vi "Lockin_Vsg_Pubudu.vi"(8 "error in (no error)":errorcluster, 11 "Transport":refnum<class "Transport.lvclass">) -> (0 "error out":errorcluster, 3 "Transport.lvclass":refnum<class "Transport.lvclass">)   [LabVIEW 2019, in "Transport.lvclass"]
uses:
  <userlib>/LevyLab/Transport/Transport/Transport.lvclass
  <userlib>/LevyLab/Transport/Control Experiment/Typedefs/Instruments--cluster.ctl
  <userlib>/LevyLab/Krohn Hite 7008/Instrument.KH7008.lvclass
  <userlib>/LevyLab/Lockin-Multichannel/Instrument.Lockin/Instrument.Lockin.lvclass
  <userlib>/LevyLab/Instrument Framework/Instrument Types/Cryostat/Instrument.Cryostat.lvclass
  <userlib>/LevyLab/Instrument Framework/Instrument Types/CBridge/Instrument.CBridge.lvclass
  <userlib>/LevyLab/Instrument Framework/Instrument Types/Delay Line/Instrument.DelayLine.lvclass
  <userlib>/LevyLab/Instrument Framework/Instrument Types/Strain/Instrument.Strain.lvclass
  <userlib>/LevyLab/Instrument Framework/Instrument Types/VNA/Instrument.VNA.lvclass
  <userlib>/LevyLab/Instrument Framework/Instrument Types/VSource/Instrument.VSource.lvclass
  <userlib>/LevyLab/Transport/Transport/Transport.lvclass/Transport.ctl
  <userlib>/LevyLab/Transport/Control Experiment/Control Experiment.lvclass/Control Experiment.ctl
  <userlib>/LevyLab/Lockin-Multichannel/Instrument.Lockin/Typedefs/Results Type--Enum.ctl
  <userlib>/LevyLab/Lockin-Multichannel/Lockin.DAQ/Typedefs/AO_Channel-Numeric.ctl
  <userlib>/LevyLab/Transport/Control Experiment/Control Experiment.lvclass
  <userlib>/LevyLab/Lockin-Multichannel/Lockin.DAQ/Lockin.DAQ.lvclass
panel:
  in  "Tab Control":enum32{"LockIn Control", "Data", "Other"}(tab)
  out "elapsed time (s)":u32=1660
  in  "Input":i32[](array[numeric])=[21]
  in  "Vmax (end)":dbl=5.0 format="%#_3p"
  in  "Vmin (start)":dbl=-5.0 format="%#_3p"
  in  "dV":dbl=0.025 format="%#_3p"
  in  "Experiment Comments":string="Vbg sweep from  0V to 100V to  -100V to 0V in steps of 0.5V\n\nstripe device:\n\nI+: 11,12,13, current mode, gain: 1000x, shunt resistor : 5kohm \nlead 12: Vac: 125uV, 7Hz, Vdc= 0mV\ndV1: 11-12 voltage mode, gain: 10x, shunt resistor : open \nVbg: 26, 1Gohm resistor\n\nhash device:\n\nI+: 16,17 current mode, gain: 1000x, shunt resistor : 5kohm \nlead 17: Vac:  5mV, 7Hz, Vdc= 0mV\n##lead 20, voltage mode, gain: 10x, shunt resistor : open \ndV1: 16-17 voltage mode, gain: 10x, shunt resistor : open \n##dV1: 16-20 voltage mode, gain: 10x, shunt resistor : open \nVbg: 26, 1Gohm resistor\n\nIn plane gates:\n3,8,15,21: 0V, 100Mohm resistors"
  in  "Experiment Folder":string="14- mega backgate sweep"
  out "T (mK)":dbl=0.001
  in  "wait after setting Vsg (ms)":u32=2000
  in  "Initial wait (ms)":u32=1000
  in  "Sweep":enum16{"Vsg", "Vbg"}(ring)
  in  "cycles (1,2,...)":i32=1 min=1 step=1
  in  "phase":dbl
  out "Field (T)":dbl=-0.0003 format="%#_13g"
  in  "function (ramp)":enum16{"Ramp", "Triangle", "Sine"}(ring)=enum."Triangle"
  in  "set \"Vsg\" to initial value?":bool
  out "time b/w points (ms)":u32=2066
  in  "stop":bool
  out "APD Signal":dbl[](graph)
  out "X Lockins":cluster{dbl[], dbl[]}[](graph)
  out "Y Lockins":cluster{dbl[], dbl[]}[](graph)
  out "G4T":cluster{dbl[], dbl[]}[](graph)
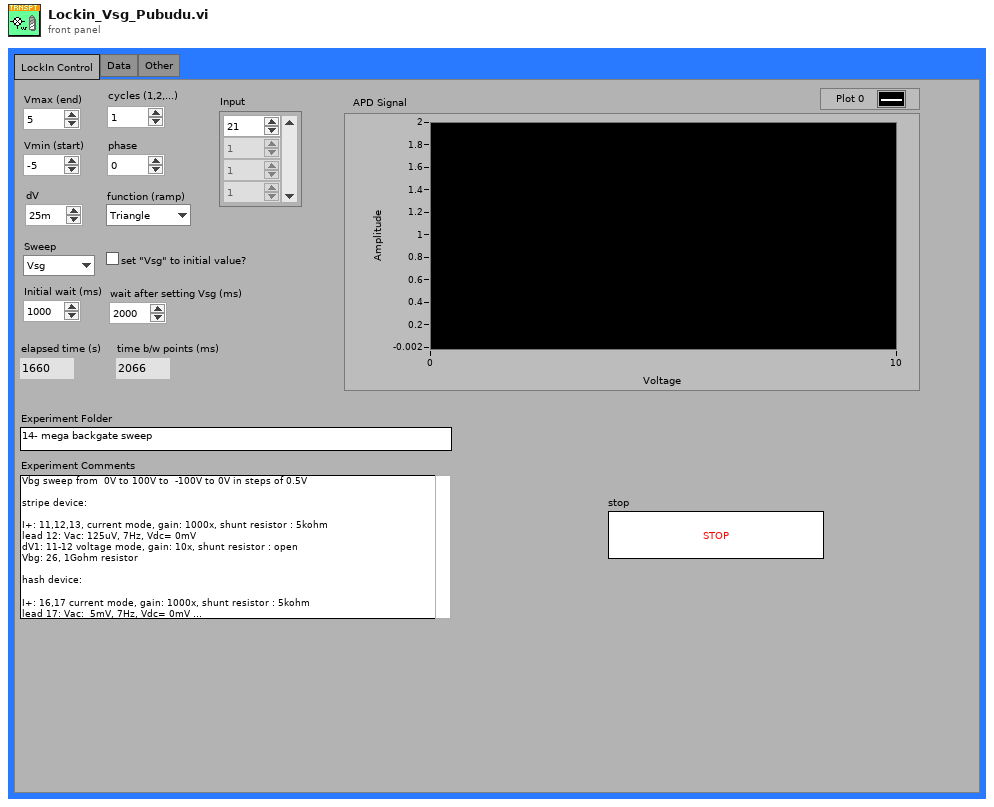
[diagram p1: front panel]
types:
  T1 = enum32{"Invalid", "Standard", "Closed", "Hidden", "Minimized", "Maximized"}
  T2 = enum32{"invalid app kind", "Development System", "Run Time System", "Student Edition", "Embedded LabVIEW", "Evaluation", "Custom"}
  T3 = typedef "Instrument.Lockin.lvclass/Results Type--Enum.ctl" = enum16{"X", "Y", "R", "Theta", "Mean"}
  T4 = typedef "Lockin.DAQ.lvclass/AO_Channel-Numeric.ctl" = i32
  T5 = typedef "Control Experiment.lvclass/Instruments--cluster.ctl" = cluster{"KH7008":refnum<class "Instrument.KH7008.lvclass">[], "Lockin":refnum<class "Instrument.Lockin.lvclass">, "Temperature":refnum<class "Instrument.Cryostat.lvclass">, "Magnet":refnum<class "Instrument.Cryostat.lvclass">, "Rotator":refnum<class "Instrument.Cryostat.lvclass">, "Level":refnum<class "Instrument.Cryostat.lvclass">, "Capacitance Bridge":refnum<class "Instrument.CBridge.lvclass">, "Delay Line":refnum<class "Instrument.DelayLine.lvclass">, "Strain Cell":refnum<class "Instrument.Strain.lvclass">, "VNA":refnum<class "Instrument.VNA.lvclass">, "Voltage Source":refnum<class "Instrument.VSource.lvclass">}
  T6 = cluster{"Core":cluster{"Current VI Reference":refnum<vi>, "Close Panel on Exit?":bool}, "Transport":refnum<class "Transport.lvclass">, "C.E.":refnum<class "Control Experiment.lvclass">, "Instruments":T5, "Sweep Values":dbl[], "Results (Dictionary)":cluster{"key":string, "value":dbl}[], "size":i32, "index":i32, "ms [0]":u32, "ms [i]":u32, "Execution:State":enum32{"Bad", "Idle", "Run top level", "Running"}}
  T7 = enum32{"Bad", "Idle", "Run top level", "Running"}
  T8 = cluster{"Current VI Reference":refnum<vi>, "Close Panel on Exit?":bool}
  T9 = cluster{"I-":i32, "I+":i32, "V1-":i32, "V1+":i32, "I2-":i32, "I2+":i32, "V2-":i32, "V2+":i32}
  T10 = typedef "Lockin.DAQ.lvclass/AO-cluster.ctl" = T11[]
  T11 = typedef "Instrument.Lockin.UI.lvclass/AO Channel--Cluster.ctl" = cluster{"Enable?":bool, "Channel":i32, "Amplitude":dbl, "Offset":dbl, "Frequency":dbl, "Phase":dbl, "Function":T12, "Sweeping?":bool}
  T12 = typedef "Lockin.DAQ.lvclass/Function-enum.ctl" = enum16{"Sine", "Triangle", "Square"}
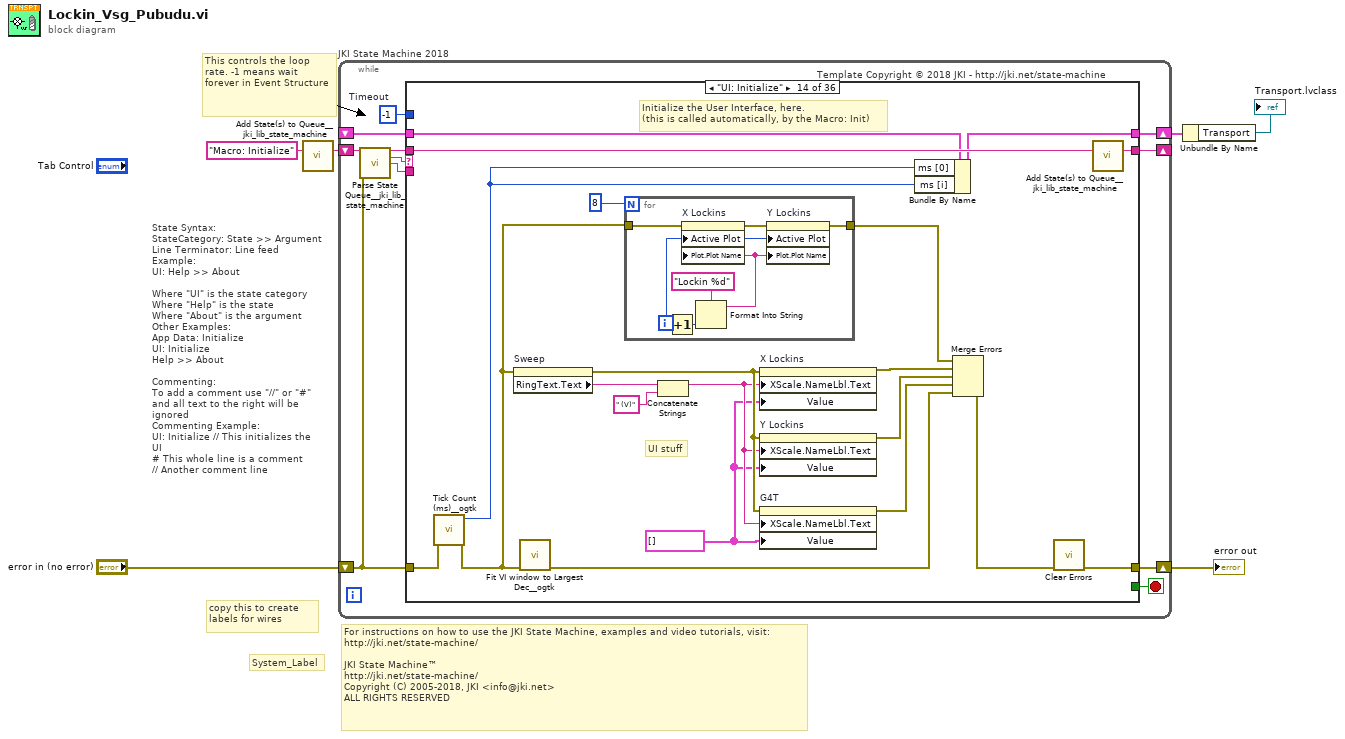
[diagram p0: block diagram]
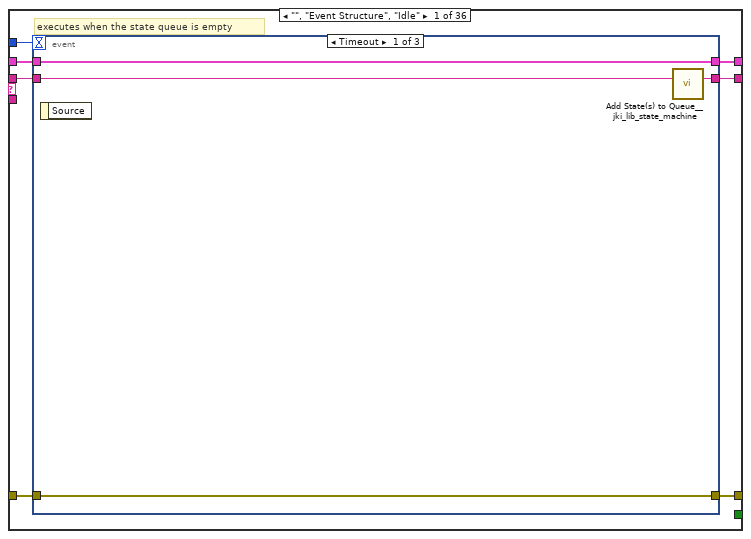
[diagram p2: hidden frame]
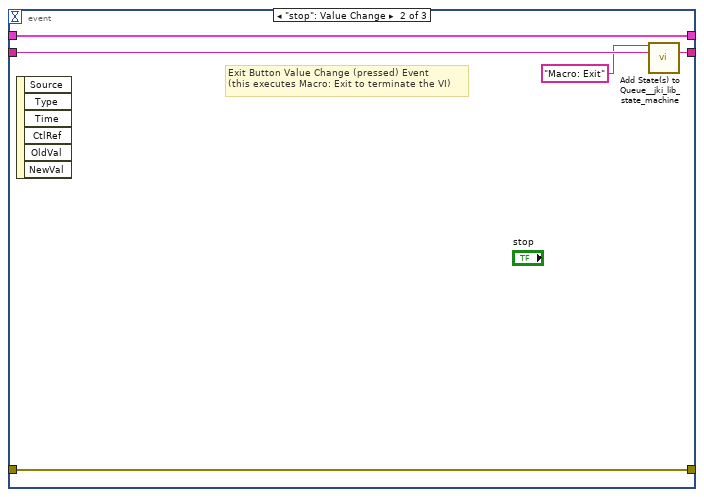
[diagram p3: hidden frame]
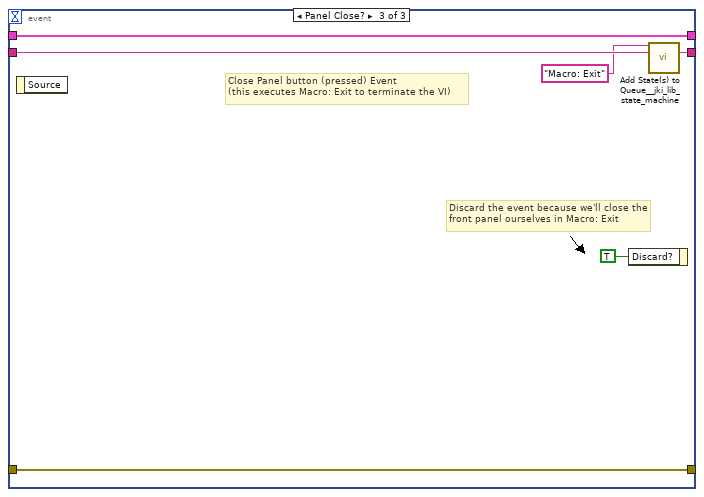
[diagram p4: hidden frame]
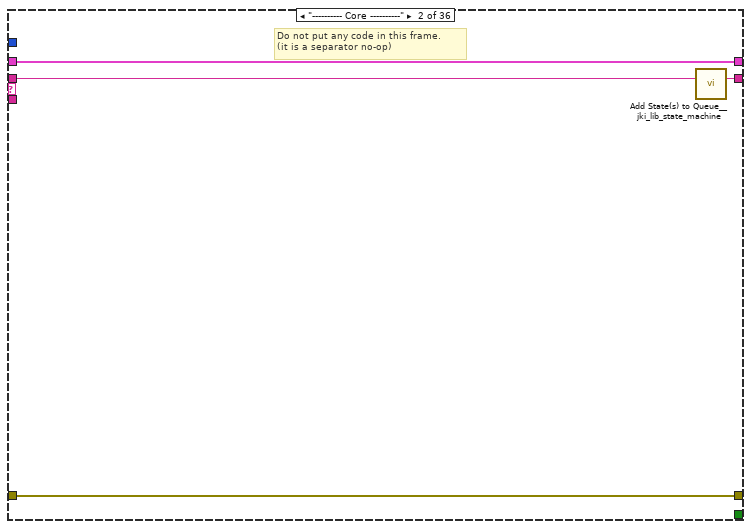
[diagram p5: hidden frame]
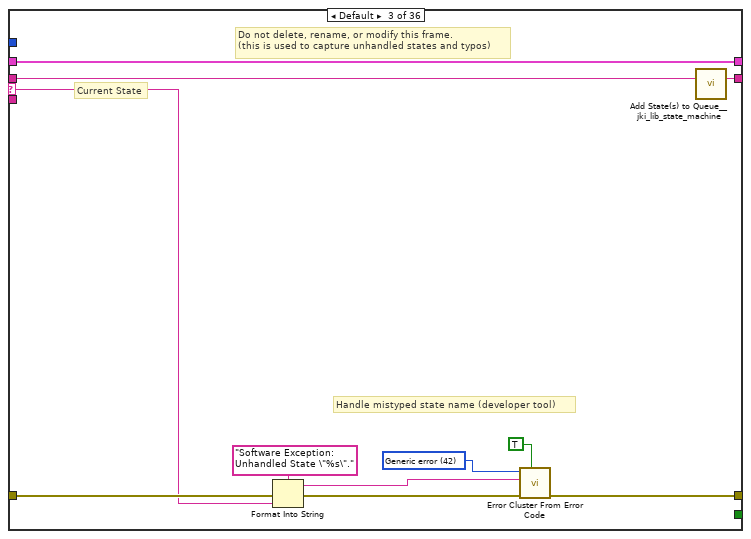
[diagram p6: hidden frame]
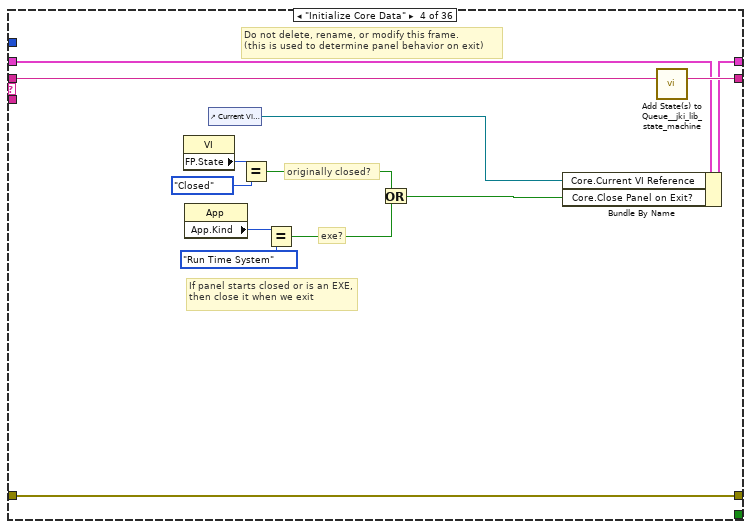
[diagram p7: hidden frame]
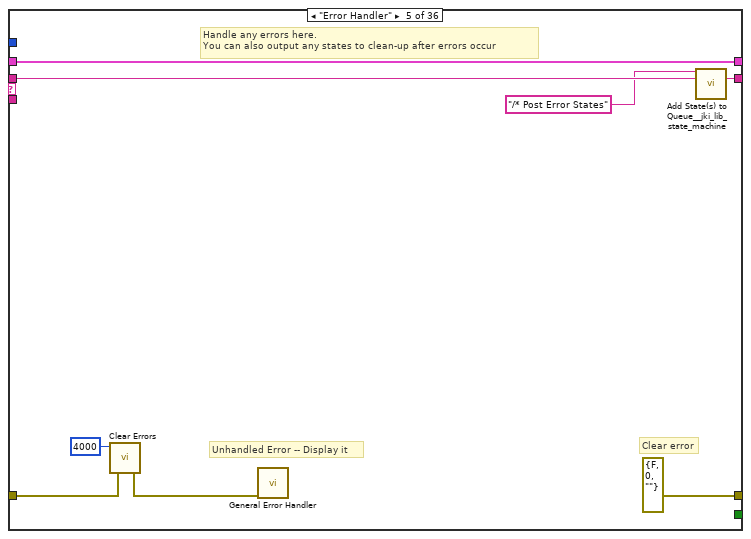
[diagram p8: hidden frame]
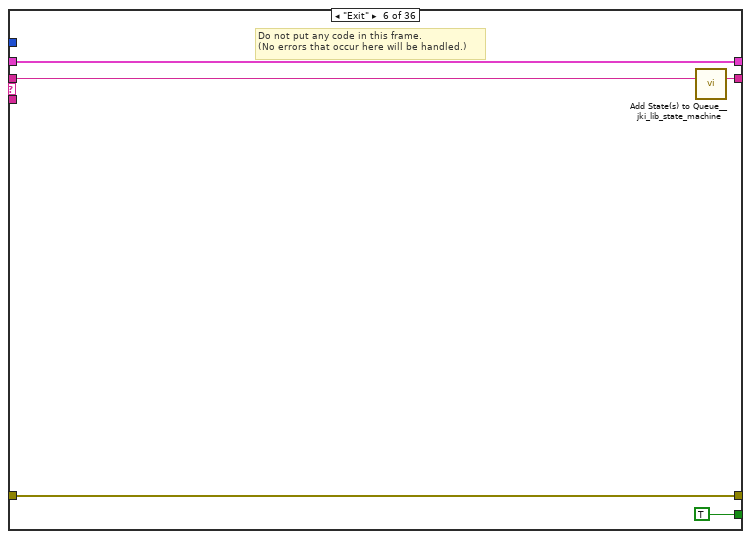
[diagram p9: hidden frame]
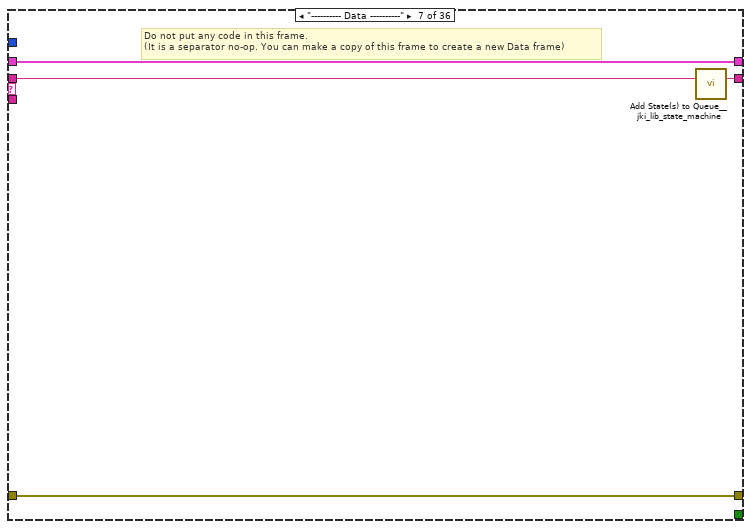
[diagram p10: hidden frame]
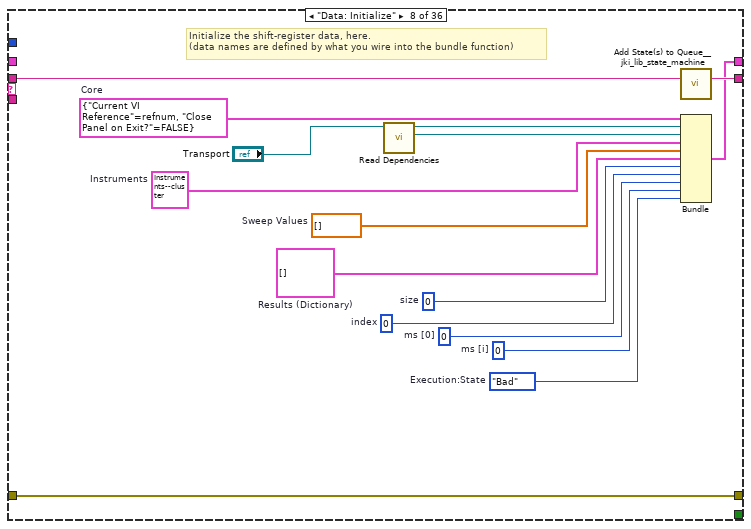
[diagram p11: hidden frame]
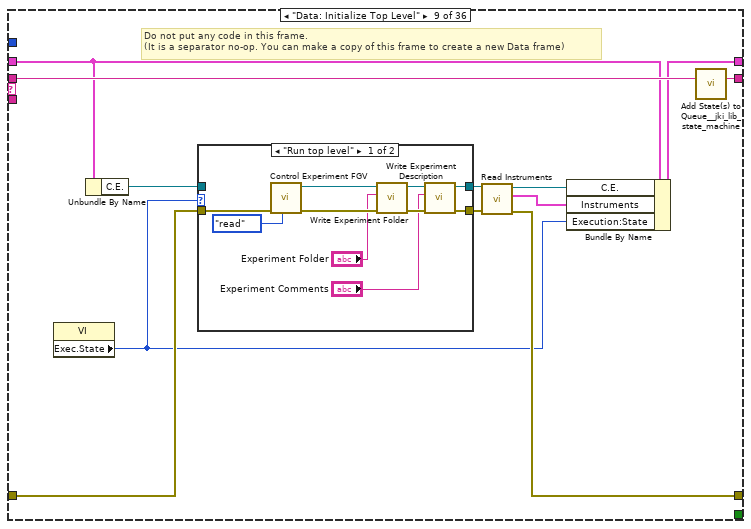
[diagram p12: hidden frame]
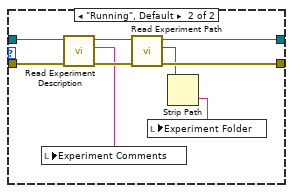
[diagram p13: hidden frame]
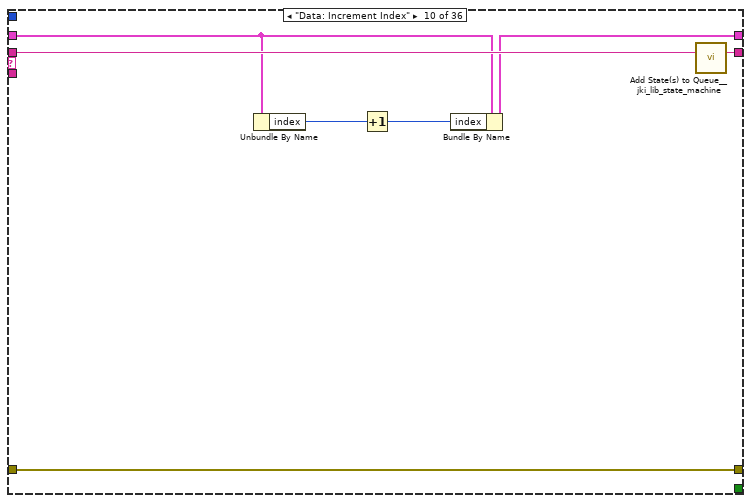
[diagram p14: hidden frame]
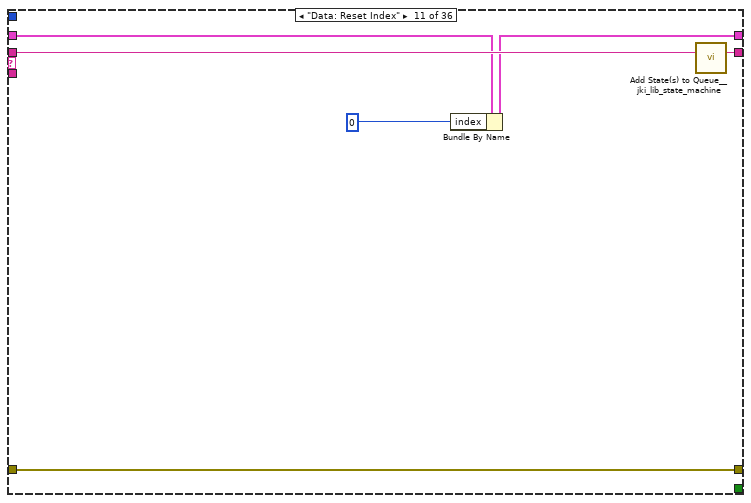
[diagram p15: hidden frame]
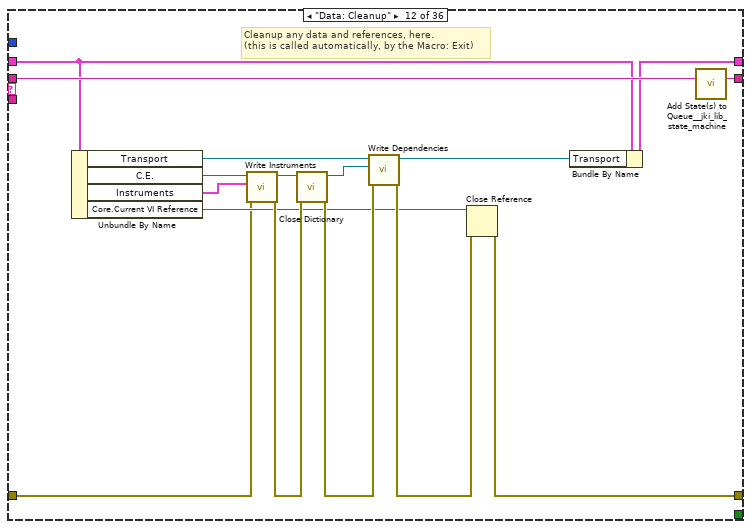
[diagram p16: hidden frame]
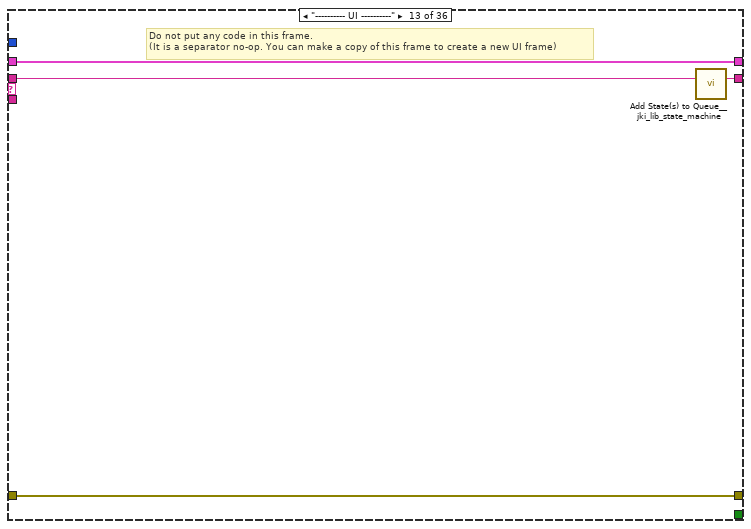
[diagram p17: hidden frame]
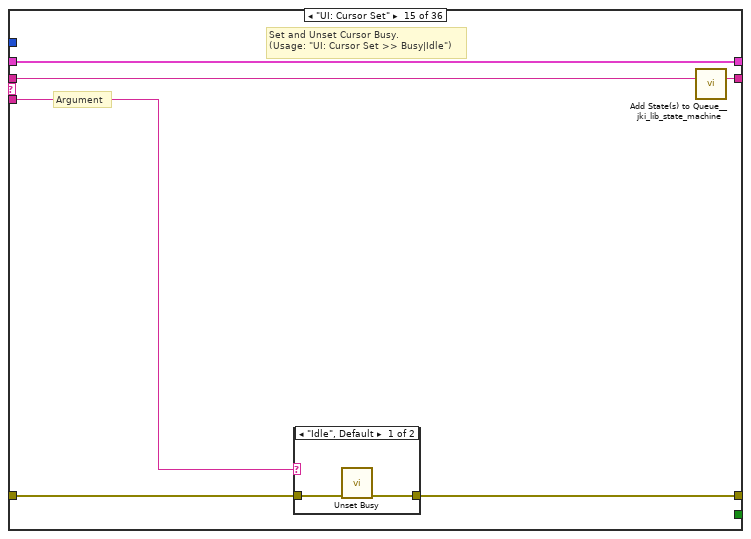
[diagram p18: hidden frame]
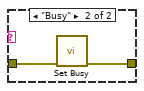
[diagram p19: hidden frame]
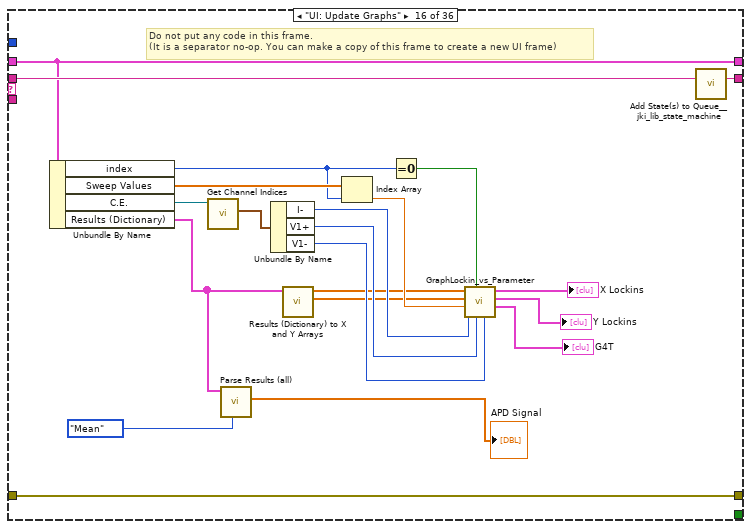
[diagram p20: hidden frame]
diagram:
  # "For instructions on how to use the JKI State Machine, examples and video tutorials, visit:\nhttp://jki.net/state-machine/\n\nJKI State Machine™\nhttp://jki.net/state-machine/\nCopyright (C) 2005-2018, JKI <info@jki.net>\nALL RIGHTS RESERVED"
  # "State Syntax:\nStateCategory: State >> Argument\nLine Terminator: Line feed\nExample:\nUI: Help >> About\n\nWhere \"UI\" is the state category\nWhere \"Help\" is the state\nWhere \"About\" is the argument\nOther Examples:\nApp Data: Initialize\nUI: Initialize\nHelp >> About\n\nCommenting:\nTo add a comment use \"//\" or \"#\" and all text to the right will be ignored\nCommenting Example:\nUI: Initialize // This initializes the UI\n# This whole line is a comment\n// Another comment line"
  # "copy this to create labels for wires"
  # "This controls the loop rate. -1 means wait forever in Event Structure"
  # "System_Label"
  n1 = call <vilib>:"Add State(s) to Queue__jki_lib_state_machine.vi"("State(s) in (\"\")"="Macro: Initialize") -> ("States Out"=w6:string)  [unwired: 14 in]
  n2 = while "JKI State Machine 2018" {
    shift-right: [w10] -> w4
    shift-left: _ -> [w9]
    shift-right: [w13] -> w2
    shift-left: "error in (no error)" -> [w7]
    shift-right: [w12] -> _
    shift-left: w6 -> [w14]
    stop <- w11 stop-if-true
    w8 = -1  # Timeout
    # "Template Copyright © 2018 JKI - http://jki.net/state-machine"
    n3 = call <vilib>:"Parse State Queue__jki_lib_state_machine.vi"("State Queue"=w14, "Error In (no error)"=w7) -> ("Remaining States"=w16:string, "Current State"=w17:string, "Arguments"=w15:string)  [unwired: 11 in]
    n4 = case shown="\"UI: Initialize\"" w17 {
      selector: w17 -> [_ _ w44 _ _ _ _ _ _ _ _ _ _ _ _ _ _ _ _ _ _ _ _ _ _ _ _ _ _ _ _ _ _ _ _ _]
      tunnel: w16 -> [w24 w43 w48 w67 w75 w80 w84 w100 w112 w138 w144 w160 w164 w184 w197 w222 w235 w242 w311 w316 w338 w348 w352 w376 w388 w395 w409 w451 w464 w477 w490 w508 w541 w545 w549 w559]
      tunnel: w15 -> [_ _ _ _ _ _ _ _ _ _ _ _ _ _ w192 _ _ w236 _ _ _ _ _ _ _ _ _ _ _ _ _ _ _ _ _ _]
      tunnel: w9 -> [w22 w40 w46 w60 w72 w78 w81 _ w103 w132 w141 w148 w161 w168 w195 w205 w230 w238 w308 w314 w331 w345 w349 w364 w385 w391 w399 w448 w460 w474 w485 w503 w537 w542 w546 w552]
      tunnel: [w21 w41 w50 w64 errorcluster {"status"=FALSE, "code"=0, "source"=""} ("error out") w77 w82 w97 w104 w136 w142 w145 w162 w173 w193 w220 w224 w239 w309 w312 w336 w346 w350 w354 w386 w392 w403 w449 w456 w468 w481 w499 w532 w543 w547 w556] -> w13
      tunnel: w7 -> [w20 w41 w49 w64 w69 w77 w82 w97 w105 w136 w142 w146 w162 w170 w194 w220 w232 w240 w309 w312 w336 w346 w350 w361 w386 w393 w402 w449 w461 w472 w482 w506 w533 w543 w547 w555]
      tunnel: [w23 w42 w47 w66 w74 w79 w83 w99 w111 w137 w143 w159 w163 w183 w196 w221 w234 w241 w310 w315 w337 w347 w351 w375 w387 w394 w408 w450 w463 w476 w489 w507 w540 w544 w548 w558] -> w12
      tunnel: [_ _ _ _ _ TRUE _ _ _ _ _ _ _ _ _ _ _ _ _ _ _ _ _ _ _ _ _ _ _ _ _ _ _ _ _ _] -> w11
      tunnel: [w19 w40 w46 w65 w72 w78 w81 w98 w102 w135 w140 w147 w161 w167 w195 w205 w229 w238 w308 w314 w331 w345 w349 w367 w385 w391 w400 w448 w459 w473 w484 w504 w538 w542 w546 w551] -> w10
      tunnel: w8 -> [w18 _ _ _ _ _ _ _ _ _ _ _ _ _ _ _ _ _ _ _ _ _ _ _ _ _ _ _ _ _ _ _ _ _ _ _]
      frame "", "Event Structure", "Idle" {
        # "executes when the state queue is empty"
        n5 = event shown="[0] Timeout" {
          selector: _ -> [_ _ _]
          dyn-events: _ -> [_ _ _]
          timeout: w18 -> [_ _ _]
          tunnel: w24 -> [w28 w33 w39]
          tunnel: [w27 w32 w38] -> w23
          tunnel: w22 -> [w25 w30 w36]
          tunnel: [w26 w31 w37] -> w21
          tunnel: w20 -> [w26 w31 w37]
          tunnel: [w25 w30 w36] -> w19
          event Timeout {
            n6 = event-data() -> ()  [unwired: 1 in, 1 out]
            n7 = call <vilib>:"Add State(s) to Queue__jki_lib_state_machine.vi"("State(s) in (\"\")"=w28) -> ("States Out"=w27:string)  [unwired: 14 in]
          }
          event "stop": Value Change {
            # "Exit Button Value Change (pressed) Event\n(this executes Macro: Exit to terminate the VI)"
            n8 = event-data() -> ()  [unwired: 1 in, 6 out]
            n9 = call <vilib>:"Add State(s) to Queue__jki_lib_state_machine.vi"("State(s) in Front (\"\")"="Macro: Exit", "State(s) in (\"\")"=w33) -> ("States Out"=w32:string)  [unwired: 13 in]
          }
          event Panel Close? {
            # "Discard the event because we'll close the front panel ourselves in Macro: Exit"
            # "Close Panel button (pressed) Event\n(this executes Macro: Exit to terminate the VI)"
            n10 = event-data() -> ()  [unwired: 1 in, 1 out]
            n11 = event-data("Discard?"=TRUE) -> ()  [unwired: 1 in, 1 out]
            n12 = call <vilib>:"Add State(s) to Queue__jki_lib_state_machine.vi"("State(s) in Front (\"\")"="Macro: Exit", "State(s) in (\"\")"=w39) -> ("States Out"=w38:string)  [unwired: 13 in]
          }
        }
      }
      frame "---------- Core ----------" {
        # "Do not put any code in this frame.\n(it is a separator no-op)"
        n13 = call <vilib>:"Add State(s) to Queue__jki_lib_state_machine.vi"("State(s) in (\"\")"=w43) -> ("States Out"=w42:string)  [unwired: 14 in]
      }
      frame Default {
        w53 = 42 items=["No error", "Argument error", "Memory is full", "Out of zone", "End of file", "File already open", "Generic file I/O error", "File not found", "File permission error", "Disk is full", "Duplicate path", "Too many files open", "System feature not enabled", "Resource file not found", "Cannot add resource", "Resource not found", "Image not found", "Image memory error", "Pen does not exist", "Config type invalid", "Config token not found", "Config parse error", "Config memory error", "Bad external code format", "Bad external code offset", "External code not present", "Null window", "Destroy window error", "Null menu", "Print aborted", "Bad print record", "Print driver error", "Windows error during printing", "Memory error during printing", "Print dialog error", "Generic print error", "Invalid device refnum", "Device not found", "Device parameter error", "Device unit error", "Cannot open device", "Device call aborted", "Generic error", "Cancelled by user", "Object ID too low", "Object ID too high", "Object not in heap", "Unknown heap", "Unknown object (invalid DefProc)", "Unknown object (DefProc not in table)", "Message out of range", "Invalid (null) method", "Unknown message", "Manager call not supported", "Bad address", "Network operation in progress", "Network operation timed out", "Connection is busy", "Network attribute not supported", "Network error", "Address in use", "System out of memory", "Connection aborted", "Connection refused", "Not connected", "Already connected", "Connection closed", "Initialization error (interapplication manager)", "Bad occurrence", "Wait on unbound occurrence handler", "Occurrence queue overflow", "Datalog type conflict", "Unused", "Unrecognized type (interapplication manager)", "Memory corrupt", "Failed to make temporary DLL", "Old CIN version", "Drag socket not found", "Failed to load drop-object", "Failed to register OLE object", "Failed to release OLE object", "Format specifier type mismatch", "Unknown format specifier", "Too few format specifiers", "Too many format specifiers", "Scan failed", "Newer CIN version", "Error converting to variant", "Runtime menu error", "Password tampered", "Variant attribute not found", "Incompatible variant data type", "Event data is not available", "Event Store is not present", "Occurrence is not found", "Event Queue is not created", "Event info is not available", "Refnum passed is NULL", "Error retrieving Class GUID", "Error retrieving CoClass GUID", "Error retrieving TypeLib GUID.", "Bad built application magic bytes.", "Specific driver is different from the specific driver associated with the Logical Name.", "There is no session opened to the class driver.", "Max Error", "MAX - Error with config objects", "MAX - Error loading configuration", "MAX - Group not supported"]
        # "Current State"
        # "Do not delete, rename, or modify this frame.\n(this is used to capture unhandled states and typos)"
        # "Handle mistyped state name (developer tool)"
        n14 = Format Into String(format string="Software Exception: Unhandled State \"%s\"." ("message"), error in=w49, w44) -> (resulting string=w52:string, error out=w51:errorcluster)  [unwired: 1 in]
        n15 = call <vilib>:"Error Cluster From Error Code.vi"("show call chain? (False)"=TRUE, "error in (no error)"=w51, "error message (\"\")"=w52, "error code (0)"=w53) -> ("error out"=w50:errorcluster)  [unwired: 5 in]
        n16 = call <vilib>:"Add State(s) to Queue__jki_lib_state_machine.vi"("State(s) in (\"\")"=w48) -> ("States Out"=w47:string)  [unwired: 14 in]
      }
      frame "Initialize Core Data" {
        # "Do not delete, rename, or modify this frame.\n(this is used to determine panel behavior on exit)"
        # "originally closed?"
        # "exe?"
        # "If panel starts closed or is an EXE, then close it when we exit"
        n17 = property class="VI"() -> ("FP.State"=w57:T1)  [unwired: 2 in, 2 out]
        n18 = property class="App"() -> ("App.Kind"=w63:T2)  [unwired: 2 in, 2 out]
        n19 = control-ref of="Current VI Reference"() -> (w58:refnum<vi>)
        n20 = Equal?(x=w57, y=T1."Closed" ("Front Panel Window:State")) -> (x = y?=w55:bool)
        n21 = Equal?(x=w63, y=T2."Run Time System" ("Application:Kind")) -> (x = y?=w61:bool)
        n22 = Or(x=w55, y=w61) -> (x .or. y?=w59:bool)
        n23 = Bundle By Name(cluster=w60, "Core.Current VI Reference"=w58, "Core.Close Panel on Exit?"=w59) -> (w65:T6)
        n24 = call <vilib>:"Add State(s) to Queue__jki_lib_state_machine.vi"("State(s) in (\"\")"=w67) -> ("States Out"=w66:string)  [unwired: 14 in]
      }
      frame "Error Handler" {
        # "Unhandled Error -- Display it"
        # "Handle any errors here.\nYou can also output any states to clean-up after errors occur"
        # "Clear error"
        n25 = call <vilib>:"Clear Errors.vi"("error in (no error)"=w69, "specific error code to clear (0: all)"=4000) -> ("error out"=w68:errorcluster)  [unwired: 4 in, 1 out]
        n26 = call <vilib>:"General Error Handler.vi"("error in (no error)"=w68) -> ()  [unwired: 10 in, 5 out]
        n27 = call <vilib>:"Add State(s) to Queue__jki_lib_state_machine.vi"("State(s) in Front (\"\")"="/* Post Error States", "State(s) in (\"\")"=w75) -> ("States Out"=w74:string)  [unwired: 13 in]
      }
      frame "Exit" {
        # "Do not put any code in this frame.\n(No errors that occur here will be handled.)"
        n28 = call <vilib>:"Add State(s) to Queue__jki_lib_state_machine.vi"("State(s) in (\"\")"=w80) -> ("States Out"=w79:string)  [unwired: 14 in]
      }
      frame "---------- Data ----------" {
        # "Do not put any code in this frame.\n(It is a separator no-op. You can make a copy of this frame to create a new Data frame)"
        n29 = call <vilib>:"Add State(s) to Queue__jki_lib_state_machine.vi"("State(s) in (\"\")"=w84) -> ("States Out"=w83:string)  [unwired: 14 in]
      }
      frame "Data: Initialize" {
        w85 = cluster{"key":string, "value":dbl}[] []  # Results (Dictionary)
        w89 = T7."Bad"  # Execution:State
        w90 = 0  # size
        w91 = u32 0  # ms [i]
        w92 = u32 0  # ms [0]
        w93 = 0  # index
        w94 = dbl[] []  # Sweep Values
        w95 = T5 {"KH7008"=[], "Lockin"=refnum, "Temperature"=refnum, "Magnet"=refnum, "Rotator"=refnum, "Level"=refnum, "Capacitance Bridge"=refnum, "Delay Line"=refnum, "Strain Cell"=refnum, "VNA"=refnum, "Voltage Source"=refnum}  # Instruments
        w96 = T8 {"Current VI Reference"=refnum, "Close Panel on Exit?"=FALSE}  # Core
        # "Initialize the shift-register data, here.\n(data names are defined by what you wire into the bundle function)"
        n30 = call <userlib>:"Read Dependencies.vi"("Transport"="Transport") -> ("C.E."=w87:refnum<class "Control Experiment.lvclass">, "Transport"=w86:refnum<class "Transport.lvclass">)  [unwired: 8 in, 1 out]
        n31 = call <vilib>:"Add State(s) to Queue__jki_lib_state_machine.vi"("State(s) in (\"\")"=w100) -> ("States Out"=w99:string)  [unwired: 14 in]
        n32 = Bundle("Core"=w96, "Transport"=w86, "C.E."=w87, "Instruments"=w95, "Sweep Values"=w94, "Results (Dictionary)"=w85, "size"=w90, "index"=w93, "ms [0]"=w92, "ms [i]"=w91, "Execution:State"=w89) -> (w98:T6)  [unwired: 1 in]
      }
      frame "Data: Initialize Top Level" {
        # "Do not put any code in this frame.\n(It is a separator no-op. You can make a copy of this frame to create a new Data frame)"
        n33 = property class="VI"() -> ("Exec.State"=w101:T7)  [unwired: 2 in, 2 out]
        n34 = Unbundle By Name(w103) -> ("C.E."=w106:refnum<class "Control Experiment.lvclass">)
        n35 = case shown="\"Run top level\"" w101 {
          tunnel: w105 -> [w122 w130]
          tunnel: [w117 w126] -> w107
          tunnel: [w116 w127] -> w108
          tunnel: w106 -> [_ w131]
          frame "Run top level" {
            n36 = call <userlib>:"Control Experiment FGV.vi"("Function"=enum16{"read", "write"}."read", "error in (no error)"=w122) -> ("error out"=w120:errorcluster, "Control Experiment.lvclass out"=w121:refnum<class "Control Experiment.lvclass">)  [unwired: 8 in]
            n37 = call <userlib>:"Write Experiment Folder.vi"("error in (no error)"=w120, "Experiment Folder"="Experiment Folder", "Control Experiment in"=w121) -> ("error out"=w118:errorcluster, "Control Experiment out"=w119:refnum<class "Control Experiment.lvclass">)  [unwired: 7 in]
            n38 = call <userlib>:"Write Experiment Description.vi"("error in (no error)"=w118, "Experiment Description"="Experiment Comments", "Control Experiment in"=w119) -> ("error out"=w117:errorcluster, "Control Experiment out"=w116:refnum<class "Control Experiment.lvclass">)  [unwired: 7 in]
          }
          frame "Running", Default {
            n39 = call <userlib>:"Read Experiment Description.vi"("error in (no error)"=w130, "Control Experiment in"=w131) -> ("error out"=w129:errorcluster, "Experiment Description"=w124:string, "Control Experiment out"=w128:refnum<class "Control Experiment.lvclass">)  [unwired: 7 in]
            n40 = local write "Experiment Comments"(w124) -> ()
            n41 = call <userlib>:"Read Experiment Path.vi"("error in (no error)"=w129, "Control Experiment in"=w128) -> ("error out"=w126:errorcluster, "Experiment Path"=w125:path, "Control Experiment out"=w127:refnum<class "Control Experiment.lvclass">)  [unwired: 7 in]
            n42 = Strip Path(path=w125) -> (name=w123:string)  [unwired: 1 out]
            n43 = local write "Experiment Folder"(w123) -> ()
          }
        }
        n44 = call <userlib>:"Read Instruments.vi"("error in (no error)"=w107, "Control Experiment in"=w108) -> ("error out"=w104:errorcluster, "Instruments"=w110:T5, "Control Experiment out"=w109:refnum<class "Control Experiment.lvclass">)  [unwired: 7 in]
        n45 = Bundle By Name(cluster=w103, "C.E."=w109, "Instruments"=w110, "Execution:State"=w101) -> (w102:T6)
        n46 = call <vilib>:"Add State(s) to Queue__jki_lib_state_machine.vi"("State(s) in (\"\")"=w112) -> ("States Out"=w111:string)  [unwired: 14 in]
      }
      frame "Data: Increment Index" {
        n47 = Unbundle By Name(w132) -> ("index"=w134:i32)
        n48 = Increment(x=w134) -> (x+1=w133:i32)
        n49 = Bundle By Name(cluster=w132, "index"=w133) -> (w135:T6)
        n50 = call <vilib>:"Add State(s) to Queue__jki_lib_state_machine.vi"("State(s) in (\"\")"=w138) -> ("States Out"=w137:string)  [unwired: 14 in]
      }
      frame "Data: Reset Index" {
        n51 = Bundle By Name(cluster=w141, "index"=0) -> (w140:T6)
        n52 = call <vilib>:"Add State(s) to Queue__jki_lib_state_machine.vi"("State(s) in (\"\")"=w144) -> ("States Out"=w143:string)  [unwired: 14 in]
      }
      frame "Data: Cleanup" {
        # "Cleanup any data and references, here.\n(this is called automatically, by the Macro: Exit)"
        n53 = Unbundle By Name(w148) -> ("Transport"=w157:refnum<class "Transport.lvclass">, "C.E."=w155:refnum<class "Control Experiment.lvclass">, "Instruments"=w153:T5, "Core.Current VI Reference"=w149:refnum<vi>)
        n54 = call <userlib>:"Write Instruments.vi"("error in (no error)"=w146, "Instruments"=w153, "Control Experiment in"=w155) -> ("error out"=w152:errorcluster, "Control Experiment out"=w154:refnum<class "Control Experiment.lvclass">)  [unwired: 7 in]
        n55 = call <userlib>:"Close Dictionary.vi"("error in (no error)"=w152, "Control Experiment in"=w154) -> ("error out"=w151:errorcluster, "Control Experiment out"=w156:refnum<class "Control Experiment.lvclass">)  [unwired: 8 in]
        n56 = call <userlib>:"Write Dependencies.vi"("error in (no error)"=w151, "Control Experiment"=w156, "Transport in"=w157) -> ("error out"=w150:errorcluster, "Transport out"=w158:refnum<class "Transport.lvclass">)  [unwired: 7 in]
        n57 = Close Reference(reference=w149, error in (no error)=w150) -> (error out=w145:errorcluster)
        n58 = Bundle By Name(cluster=w148, "Transport"=w158) -> (w147:T6)
        n59 = call <vilib>:"Add State(s) to Queue__jki_lib_state_machine.vi"("State(s) in (\"\")"=w160) -> ("States Out"=w159:string)  [unwired: 14 in]
      }
      frame "---------- UI ----------" {
        # "Do not put any code in this frame.\n(It is a separator no-op. You can make a copy of this frame to create a new UI frame)"
        n60 = call <vilib>:"Add State(s) to Queue__jki_lib_state_machine.vi"("State(s) in (\"\")"=w164) -> ("States Out"=w163:string)  [unwired: 14 in]
      }
      frame "UI: Initialize" {
        w165 = cluster{dbl[], dbl[]}[] [] ("G4T")
        # "UI stuff"
        # "Initialize the User Interface, here.\n(this is called automatically, by the Macro: Init)"
        n61 = call <userlib>:"Tick Count (ms)__ogtk.vi"("error in (no error)"=w170) -> ("error out"=w169:errorcluster, "millisecond timer value"=w166:u32)  [unwired: 9 in]
        n62 = property on="Sweep" class="Enum (strict)"(error in=w169) -> (error out=w178:errorcluster, "RingText.Text"=w176:string)  [unwired: 1 in, 1 out]
        n63 = call <userlib>:"Fit VI window to Largest Dec__ogtk.vi"("error in (no error)"=w169) -> ("error out"=w172:errorcluster)  [unwired: 5 in, 1 out]
        n64 = for {
          N: 8 -> [_]
          tunnel: [w185] -> w179
          tunnel: w169 -> [w190]
          i -> [w188]
          n65 = Increment(x=w188) -> (x+1=w186:i32)
          n66 = Format Into String(format string="Lockin %d", w186) -> (resulting string=w189:string)  [unwired: 2 in, 1 out]
          n67 = property on="X Lockins" class="XYGraph (strict)"(error in=w190, "Active Plot"=w188, "Plot.Plot Name"=w189) -> (error out=w187:errorcluster)  [unwired: 1 in, 1 out]
          n68 = property on="Y Lockins" class="XYGraph (strict)"(error in=w187, "Active Plot"=w188, "Plot.Plot Name"=w189) -> (error out=w185:errorcluster)  [unwired: 1 in, 1 out]
        }
        n69 = Concatenate Strings(w176, " (V)" ("string")) -> (w177:string)
        n70 = property on="X Lockins" class="XYGraph (strict)"(error in=w178, "XScale.NameLbl.Text"=w177, "Value"=w165) -> (error out=w180:errorcluster)  [unwired: 1 in, 1 out]
        n71 = property on="Y Lockins" class="XYGraph (strict)"(error in=w178, "XScale.NameLbl.Text"=w177, "Value"=w165) -> (error out=w181:errorcluster)  [unwired: 1 in, 1 out]
        n72 = property on="G4T" class="XYGraph (strict)"(error in=w178, "XScale.NameLbl.Text"=w177, "Value"=w165) -> (error out=w182:errorcluster)  [unwired: 1 in, 1 out]
        n73 = Bundle By Name(cluster=w168, "ms [0]"=w166, "ms [i]"=w166) -> (w167:T6)
        n74 = Merge Errors(w179, w180, w181, w182, w172) -> (w171:errorcluster)
        n75 = call <vilib>:"Clear Errors.vi"("error in (no error)"=w171) -> ("error out"=w173:errorcluster)  [unwired: 5 in, 1 out]
        n76 = call <vilib>:"Add State(s) to Queue__jki_lib_state_machine.vi"("State(s) in (\"\")"=w184) -> ("States Out"=w183:string)  [unwired: 14 in]
      }
      frame "UI: Cursor Set" {
        # "Argument"
        # "Set and Unset Cursor Busy.\n(Usage: \"UI: Cursor Set >> Busy|Idle\")"
        n77 = case shown="\"Idle\", Default" w192 {
          tunnel: w194 -> [w199 w201]
          tunnel: [w198 w200] -> w193
          frame "Idle", Default {
            n78 = call <vilib>:"Unset Busy.vi"("error in (no error)"=w199) -> ("error out"=w198:errorcluster)  [unwired: 10 in]
          }
          frame "Busy" {
            n79 = call <vilib>:"Set Busy.vi"("error in (no error)"=w201) -> ("error out"=w200:errorcluster)  [unwired: 9 in, 1 out]
          }
        }
        n80 = call <vilib>:"Add State(s) to Queue__jki_lib_state_machine.vi"("State(s) in (\"\")"=w197) -> ("States Out"=w196:string)  [unwired: 14 in]
      }
      frame "UI: Update Graphs" {
        # "Do not put any code in this frame.\n(It is a separator no-op. You can make a copy of this frame to create a new UI frame)"
        n81 = Unbundle By Name(w205) -> ("index"=w208:i32, "Sweep Values"=w211:dbl[], "C.E."=w218:refnum<class "Control Experiment.lvclass">, "Results (Dictionary)"=w204:cluster{"key":string, "value":dbl}[])
        n82 = call <userlib>:"Get Channel Indices.vi"("Control Experiment in"=w218) -> ("Indices"=w217:T9)  [unwired: 8 in, 2 out]
        n83 = call <userlib>:"Parse Results (all).vi"("Type"=Results_Type--Enum."Mean", "Results (Dictionary)"=w204) -> ("Data"=→"APD Signal":dbl[])  [unwired: 6 in, 3 out]
        n84 = Unbundle By Name(w217) -> ("I-"=w214:i32, "V1+"=w216:i32, "V1-"=w215:i32)
        n85 = call <userlib>:"Results (Dictionary) to X and Y Arrays.vi"("Results (Dictionary)"=w204) -> ("Y"=w206:dbl[], "X"=w207:dbl[])  [unwired: 9 in]
        n86 = Index Array(array=w211, index=w208) -> (element=w210:dbl)
        n87 = Equal To 0?(x=w208) -> (x = 0?=w209:bool)
        n88 = call <userlib>:"GraphLockin_vs_Parameter.vi"("V-"=w215, "V+"=w216, "reset?"=w209, "Current"=w214, "Parameter"=w210, "Y [ ]"=w206, "X[ ]"=w207) -> ("G(e2/h) vs Parameter"=→"G4T":cluster{"Y":dbl[], "Y":dbl[]}[], "Y vs Parameter"=→"Y Lockins":cluster{dbl[], dbl[]}[], "X vs Parameter"=→"X Lockins":cluster{dbl[], dbl[]}[])  [unwired: 1 in, 1 out]
        n89 = call <vilib>:"Add State(s) to Queue__jki_lib_state_machine.vi"("State(s) in (\"\")"=w222) -> ("States Out"=w221:string)  [unwired: 14 in]
      }
      frame "UI: Update Timer" {
        n90 = Unbundle By Name(w230) -> ("ms [0]"=w231:u32)
        n91 = call <userlib>:"Tick Count (ms)__ogtk.vi"("error in (no error)"=w232) -> ("error out"=w225:errorcluster, "millisecond timer value"=w223:u32)  [unwired: 9 in]
        n92 = Subtract(x=w223, y=w231) -> (x-y=w227:u32)
        n93 = call <userlib>:"MGI Milliseconds Since Last Call.vi"("Error In"=w225) -> ("ms"=→"time b/w points (ms)":u32, "Error Out"=w224:errorcluster)  [unwired: 5 in]
        n94 = Divide(x=w227, y=u32 1000 ("x")) -> (x/y=→"elapsed time (s)":dbl)
        n95 = Bundle By Name(cluster=w230, "ms [i]"=w223) -> (w229:T6)
        n96 = call <vilib>:"Add State(s) to Queue__jki_lib_state_machine.vi"("State(s) in (\"\")"=w235) -> ("States Out"=w234:string)  [unwired: 14 in]
      }
      frame "UI: Front Panel State" {
        # "Argument"
        # "Set Front Panel Open or Closed\n(Usage: \"UI: Front Panel State >> Open|Close\")"
        n97 = Unbundle By Name(w238) -> ("Core.Current VI Reference"=w237:refnum<vi>)
        n98 = case shown="\"Minimize\", \"Minimized\"" w236 {
          tunnel: w240 -> [w248 w263 w274 w287 w300]
          tunnel: [w250 w264 w276 w289 w302] -> w239
          tunnel: w237 -> [w249 w261 w275 w288 w301]
          frame "Open", "Standard", Default {
            w243 = T1."Standard" ("State")
            n99 = property class="VI"(reference=w249, error in=w248) -> (reference out=w246:refnum<vi>, error out=w247:errorcluster, "FP.State"=w245:T1)
            n100 = Not Equal?(x=w245, y=w243) -> (x != y?=w244:bool)
            n101 = case shown="True" w244 {
              tunnel: [w254 w256] -> w250
              tunnel: w247 -> [w253 w256]
              tunnel: w246 -> [w252 _]
              tunnel: w243 -> [w251 _]
              frame True {
                n102 = invoke class="VI" method="FP.Open"(reference=w252, error in=w253, "Activate"=TRUE, "State"=w251) -> (error out=w254:errorcluster)  [unwired: 1 in, 4 out]
              }
              frame False {
              }
            }
          }
          frame "Close", "Closed" {
            n103 = property class="VI"(reference=w261, error in=w263) -> (reference out=w260:refnum<vi>, error out=w262:errorcluster, "FP.State"=w258:T1)
            n104 = Not Equal?(x=w258, y=T1."Closed" ("Front Panel Window:State")) -> (x != y?=w257:bool)
            n105 = case shown="True" w257 {
              tunnel: [w265 w268] -> w264
              tunnel: w262 -> [w265 w267]
              tunnel: w260 -> [_ w266]
              frame False {
              }
              frame True {
                n106 = invoke class="VI" method="FP.Close"(reference=w266, error in=w267) -> (error out=w268:errorcluster)  [unwired: 1 in, 2 out]
              }
            }
          }
          frame "Hidden", "Hide" {
            w269 = T1."Hidden" ("State")
            n107 = property class="VI"(reference=w275, error in=w274) -> (reference out=w272:refnum<vi>, error out=w273:errorcluster, "FP.State"=w271:T1)
            n108 = Not Equal?(x=w271, y=w269) -> (x != y?=w270:bool)
            n109 = case shown="True" w270 {
              tunnel: [w280 w281] -> w276
              tunnel: w273 -> [w279 w281]
              tunnel: w272 -> [w278 _]
              tunnel: w269 -> [w277 _]
              frame True {
                n110 = invoke class="VI" method="FP.Open"(reference=w278, error in=w279, "State"=w277) -> (error out=w280:errorcluster)  [unwired: 2 in, 4 out]
              }
              frame False {
              }
            }
          }
          frame "Minimize", "Minimized" {
            w282 = T1."Minimized" ("State")
            n111 = property class="VI"(reference=w288, error in=w287) -> (reference out=w285:refnum<vi>, error out=w286:errorcluster, "FP.State"=w284:T1)
            n112 = Not Equal?(x=w284, y=w282) -> (x != y?=w283:bool)
            n113 = case shown="True" w283 {
              tunnel: [w293 w294] -> w289
              tunnel: w286 -> [w292 w294]
              tunnel: w285 -> [w291 _]
              tunnel: w282 -> [w290 _]
              frame True {
                n114 = invoke class="VI" method="FP.Open"(reference=w291, error in=w292, "State"=w290) -> (error out=w293:errorcluster)  [unwired: 2 in, 4 out]
              }
              frame False {
              }
            }
          }
          frame "Maximize", "Maximized" {
            w295 = T1."Maximized" ("State")
            n115 = property class="VI"(reference=w301, error in=w300) -> (reference out=w298:refnum<vi>, error out=w299:errorcluster, "FP.State"=w297:T1)
            n116 = Not Equal?(x=w297, y=w295) -> (x != y?=w296:bool)
            n117 = case shown="True" w296 {
              tunnel: [w306 w307] -> w302
              tunnel: w299 -> [w305 w307]
              tunnel: w298 -> [w304 _]
              tunnel: w295 -> [w303 _]
              frame True {
                n118 = invoke class="VI" method="FP.Open"(reference=w304, error in=w305, "State"=w303) -> (error out=w306:errorcluster)  [unwired: 2 in, 4 out]
              }
              frame False {
              }
            }
          }
        }
        n119 = call <vilib>:"Add State(s) to Queue__jki_lib_state_machine.vi"("State(s) in (\"\")"=w242) -> ("States Out"=w241:string)  [unwired: 14 in]
      }
      frame "---------- Macro ----------" {
        # "Do not put any code in this frame.\n(It is a separator no-op. You can make a copy of this frame to create a new Macro frame)"
        n120 = call <vilib>:"Add State(s) to Queue__jki_lib_state_machine.vi"("State(s) in (\"\")"=w311) -> ("States Out"=w310:string)  [unwired: 14 in]
      }
      frame "Macro: Initialize" {
        # "Initialization Macro\n(This is called once, when the VI starts)"
        n121 = call <vilib>:"Add State(s) to Queue__jki_lib_state_machine.vi"("State(s) in Front (\"\")"="Data: Initialize\nInitialize Core Data\nUI: Initialize\nUI: Front Panel State >> Open\nData: Initialize Top Level\nData: Reset Index\nMeasure: Temperature\nMeasure: Magnet\nMeasure: Capacitance\nSweep: Initialize\nMacro: Sweep", "State(s) in (\"\")"=w316) -> ("States Out"=w315:string)  [unwired: 13 in]
      }
      frame "Macro: Sweep" {
        # "stop if true"
        # "continue if true"
        # "sweep is finished"
        # "keep sweeping"
        # "Do not put any code in this frame.\n(It is a separator no-op. You can make a copy of this frame to create a new Macro frame)"
        n122 = Unbundle By Name(w331) -> ("size"=w332:i32, "index"=w335:i32)
        n123 = Decrement(x=w332) -> (x-1=w325:i32)
        n124 = local read "stop"() -> (w318:bool)
        n125 = Not Equal?(x=w325, y=w335) -> (x != y?=w320:bool)
        n126 = Not(x=w318) -> (.not. x?=w319:bool)
        n127 = And(x=w319, y=w320) -> (x .and. y?=w317:bool)
        n128 = Select(t="Data: Reset Index\nConfigure: Set" ("State(s) in Front (\"\")"), s="set \"Vsg\" to initial value?", f="" ("State(s) in Front (\"\")")) -> (s? t:f=w322:string)
        n129 = call <vilib>:"Add State(s) to Queue__jki_lib_state_machine.vi"("State(s) in Front (\"\")"="File: Save" ("State(s) in Front (\"\")"), "State(s) in (\"\")"=w322, "State(s) at Back (\"\")"="Macro: Exit" ("State(s) in Front (\"\")")) -> ("States Out"=w326:string)  [unwired: 12 in]
        n130 = Select(t="Macro: Sweep" ("State(s) in Front (\"\")"), s=w317, f=w326) -> (s? t:f=w334:string)
        n131 = call <vilib>:"Add State(s) to Queue__jki_lib_state_machine.vi"("State(s) in Front (\"\")"="Configure: Set\nConfigure: Wait\nMeasure: Lockin\nMeasure: Time\n//Measure: Temperature\nUI: Update Graphs\nUI: Update Timer\nData: Increment Index" ("State(s) in Front (\"\")"), "State(s) at Back (\"\")"=w334) -> ("States Out"=w324:string)  [unwired: 13 in]
        n132 = call <vilib>:"Add State(s) to Queue__jki_lib_state_machine.vi"("State(s) in (\"\")"=w338, "State(s) at Back (\"\")"=w324) -> ("States Out"=w337:string)  [unwired: 13 in]
      }
      frame "Macro: Exit" {
        # "Exit Macro\n(This is called once, when the VI exits)"
        n133 = Unbundle By Name(w345) -> ("Core.Close Panel on Exit?"=w344:bool)
        n134 = Select(t="UI: Front Panel State >> Close", s=w344, f="") -> (s? t:f=w341:string)
        n135 = call <vilib>:"Add State(s) to Queue__jki_lib_state_machine.vi"("State(s) in (\"\")"=w341, "State(s) at Back (\"\")"="Data: Cleanup\nExit") -> ("States Out"=w339:string)  [unwired: 13 in]
        n136 = call <vilib>:"Add State(s) to Queue__jki_lib_state_machine.vi"("State(s) in Front (\"\")"=w339, "State(s) in (\"\")"=w348) -> ("States Out"=w347:string)  [unwired: 13 in]
      }
      frame "---------- Sweep ----------" {
        # "Do not put any code in this frame.\n(It is a separator no-op. You can make a copy of this frame to create a new Macro frame)"
        n137 = call <vilib>:"Add State(s) to Queue__jki_lib_state_machine.vi"("State(s) in (\"\")"=w352) -> ("States Out"=w351:string)  [unwired: 14 in]
      }
      frame "Sweep: Initialize" {
        # "define sweep"
        # "Do not put any code in this frame.\n(It is a separator no-op. You can make a copy of this frame to create a new Macro frame)"
        n138 = Unbundle By Name(w364) -> ("C.E."=w363:refnum<class "Control Experiment.lvclass">)
        n139 = call <userlib>:"Max_Min_conversion.vi"("Min"="Vmin (start)", "Max"="Vmax (end)") -> ("offset"=w369:dbl, "Amplitude"=w368:dbl)  [unwired: 8 in]
        n140 = local read "Sweep"() -> (w353:enum16{"Vsg", "Vbg"})
        n141 = local read "Input"() -> (w356:i32[])
        n142 = call <userlib>:"Ramp.vi"("phase"="phase", "function (ramp)"="function (ramp)", "cycles (1,2,...)"="cycles (1,2,...)", "step size"="dV", "offset"=w369, "amplitude"=w368) -> ("Waveform Graph"=w365:dbl[])  [unwired: 3 in, 2 out]
        n143 = Format Into String(error in=w361, w353) -> (resulting string=w359:string, error out=w360:errorcluster)  [unwired: 2 in]
        n144 = call <userlib>:"Write Dictionary Element.vi"("error in (no error)"=w360, "value"=w365, "key"=w359, "Control Experiment in"=w363) -> ("error out"=w355:errorcluster, "Control Experiment out"=w358:refnum<class "Control Experiment.lvclass">)  [unwired: 6 in]
        n145 = case shown="\"Vsg\", Default" w353 {
          tunnel: w358 -> [w378 w384]
          tunnel: [w378 w383] -> w357
          tunnel: w356 -> [_ w382]
          tunnel: w355 -> [w377 w380]
          tunnel: [w377 w379] -> w354
          frame "Vbg" {
          }
          frame "Vsg", Default {
            n146 = call <userlib>:"Write Dictionary Element.vi"("error in (no error)"=w380, "value"=w382, "key"="Sweep Channels", "Control Experiment in"=w384) -> ("error out"=w379:errorcluster, "Control Experiment out"=w383:refnum<class "Control Experiment.lvclass">)  [unwired: 6 in]
          }
        }
        n147 = Array Size(array=w365) -> (size(s)=w362:i32)
        n148 = Bundle By Name(cluster=w364, "Sweep Values"=w365, "size"=w362, "C.E."=w357) -> (w367:T6)
        n149 = call <vilib>:"Add State(s) to Queue__jki_lib_state_machine.vi"("State(s) in (\"\")"=w376) -> ("States Out"=w375:string)  [unwired: 14 in]
      }
      frame "---------- Configure ----------" {
        # "Do not put any code in this frame.\n(It is a separator no-op. You can make a copy of this frame to create a new Macro frame)"
        n150 = call <vilib>:"Add State(s) to Queue__jki_lib_state_machine.vi"("State(s) in (\"\")"=w388) -> ("States Out"=w387:string)  [unwired: 14 in]
      }
      frame "Configure: Wait" {
        # "Do not put any code in this frame.\n(It is a separator no-op. You can make a copy of this frame to create a new Macro frame)"
        n151 = Unbundle By Name(w391) -> ("index"=w390:i32)
        n152 = case shown="Default" w390 {
          tunnel: ["Initial wait (ms)" "wait after setting Vsg (ms)"] -> w389
          frame 0 {
          }
          frame Default {
          }
        }
        n153 = call <userlib>:"Wait (ms)__ogtk.vi"("error in (no error)"=w393, "milliseconds to wait"=w389) -> ("error out"=w392:errorcluster)  [unwired: 8 in, 1 out]
        n154 = call <vilib>:"Add State(s) to Queue__jki_lib_state_machine.vi"("State(s) in (\"\")"=w395) -> ("States Out"=w394:string)  [unwired: 14 in]
      }
      frame "Configure: Set" {
        # "do this instead of \nJSON file"
        # "Do not put any code in this frame.\n(It is a separator no-op. You can make a copy of this frame to create a new Macro frame)"
        n155 = Unbundle By Name(w399) -> ("Instruments.Lockin"=w407:refnum<class "Instrument.Lockin.lvclass">, "Sweep Values"=w406:dbl[], "index"=w405:i32)
        n156 = Index Array(array=w406, index=w405) -> (element=w401:dbl)
        n157 = case shown="\"Vsg\", Default" "Sweep" {
          tunnel: w407 -> [w413 w447]
          tunnel: w402 -> [w418 w446]
          tunnel: w401 -> [w415 w443]
          tunnel: [w417 w444] -> w403
          tunnel: [w411 w442] -> w398
          frame "Vsg", Default {
            n158 = call <userlib>:"getAOconfig.vi"("Instrument.Lockin in"=w413) -> ("AOconfig"=w416:T10)  [unwired: 8 in, 2 out]
            n159 = Decrement(x="Input") -> (x-1=w412:i32[])
            n160 = for {
              tunnel: w415 -> [w440]
              shift-right: [w436] -> w410
              shift-left: w416 -> [w438]
              tunnel: w412 -> [w437] mode=indexing
              n161 = Index Array(array=w438, index=w437) -> (element=w441:T11)
              n162 = Bundle By Name(cluster=w441, "Offset"=w440) -> (w439:T11)
              n163 = Replace Array Subset(array=w438, new element=w439, index=w437) -> (w436:T10)
            }
            n164 = disable-structure shown="Enabled" {
              disable-tunnel: w418 -> [w424 w432]
              disable-tunnel: [w423 w431] -> w417
              disable-tunnel: w415 -> [w422 _]
              disable-tunnel: "Input" -> [w421 _]
              disable-tunnel: w413 -> [w420 w434]
              disable-tunnel: [w419 w433] -> w411
              disable-tunnel: w410 -> [_ w435]
              frame Disabled {
                n165 = for {
                  tunnel: w421 -> [w426] mode=indexing
                  tunnel: w422 -> [w425]
                  tunnel: w424 -> [w429]
                  tunnel: [w428] -> w423
                  shift-right: [w427] -> w419
                  shift-left: w420 -> [w430]
                  n166 = call <userlib>:"setAO_DC.vi"("error in (no error)"=w429, "DC (V)"=w425, "AO Channel"=w426, "Instrument.Lockin in"=w430) -> ("error out"=w428:errorcluster, "Instrument.Lockin out"=w427:refnum<class "Instrument.Lockin.lvclass">)  [unwired: 6 in]
                }
              }
              frame Enabled {
                n167 = call <userlib>:"setAO.vi"("error in (no error)"=w432, "Channels: AO"=w435, "Instrument.Lockin in"=w434) -> ("error out"=w431:errorcluster, "Instrument.Lockin out"=w433:refnum<class "Instrument.Lockin.lvclass">)  [unwired: 7 in]
              }
            }
          }
          frame "Vbg" {
            n168 = call <userlib>:"setAUX.vi"("error in (no error)"=w446, "AUX (V)"=w443, "Channel"=T4 1, "Instrument.Lockin in"=w447) -> ("error out"=w444:errorcluster, "Instrument.Lockin out"=w442:refnum<class "Instrument.Lockin.lvclass">)  [unwired: 6 in]
          }
        }
        n169 = Bundle By Name(cluster=w399, "Instruments.Lockin"=w398) -> (w400:T6)
        n170 = call <vilib>:"Add State(s) to Queue__jki_lib_state_machine.vi"("State(s) in (\"\")"=w409) -> ("States Out"=w408:string)  [unwired: 14 in]
      }
      frame "---------- Measure ----------" {
        # "Template Separator\n(You can make a copy of, or modify, this frame)"
        n171 = call <vilib>:"Add State(s) to Queue__jki_lib_state_machine.vi"("State(s) in (\"\")"=w451) -> ("States Out"=w450:string)  [unwired: 14 in]
      }
      frame "Measure: Temperature" {
        # "Your code here.\n(You can make a copy of, or modify, this frame)"
        n172 = Unbundle By Name(w460) -> ("C.E."=w455:refnum<class "Control Experiment.lvclass">, "Instruments.Temperature"=w462:refnum<class "Instrument.Cryostat.lvclass">)
        n173 = call-dynamic "Get Temperature.vi"("error in (no error)"=w461, "Instrument.Cryostat in"=w462) -> ("error out"=w457:errorcluster, "Temperature (K)"=w453:dbl, "Instrument.Cryostat out"=w452:refnum<class "Instrument.Cryostat.lvclass">)  [unwired: 5 in, 2 out]
        "T (mK)" <- w453
        n174 = call <userlib>:"Write Dictionary Element.vi"("error in (no error)"=w457, "value"=w453, "key"="Temperature", "Control Experiment in"=w455) -> ("error out"=w456:errorcluster, "Control Experiment out"=w454:refnum<class "Control Experiment.lvclass">)  [unwired: 6 in]
        n175 = Bundle By Name(cluster=w460, "Instruments.Temperature"=w452, "C.E."=w454) -> (w459:T6)
        n176 = call <vilib>:"Add State(s) to Queue__jki_lib_state_machine.vi"("State(s) in (\"\")"=w464) -> ("States Out"=w463:string)  [unwired: 14 in]
      }
      frame "Measure: Magnet" {
        # "Your code here.\n(You can make a copy of, or modify, this frame)"
        n177 = Unbundle By Name(w474) -> ("C.E."=w470:refnum<class "Control Experiment.lvclass">, "Instruments.Magnet"=w475:refnum<class "Instrument.Cryostat.lvclass">)
        n178 = call-dynamic "Get Magnet.vi"("error in (no error)"=w472, "Instrument.Cryostat in"=w475) -> ("error out"=w467:errorcluster, "B Field (T)"=w469:dbl, "Instrument.Cryostat out"=w466:refnum<class "Instrument.Cryostat.lvclass">)  [unwired: 5 in, 2 out]
        "Field (T)" <- w469
        n179 = call <userlib>:"Write Dictionary Element.vi"("error in (no error)"=w467, "value"=w469, "key"="Magnet", "Control Experiment in"=w470) -> ("error out"=w468:errorcluster, "Control Experiment out"=w471:refnum<class "Control Experiment.lvclass">)  [unwired: 6 in]
        n180 = Bundle By Name(cluster=w474, "Instruments.Magnet"=w466, "C.E."=w471) -> (w473:T6)
        n181 = call <vilib>:"Add State(s) to Queue__jki_lib_state_machine.vi"("State(s) in (\"\")"=w477) -> ("States Out"=w476:string)  [unwired: 14 in]
      }
      frame "Measure: Capacitance" {
        # "Your code here.\n(You can make a copy of, or modify, this frame)"
        n182 = Unbundle By Name(w485) -> ("C.E."=w486:refnum<class "Control Experiment.lvclass">, "Instruments.Capacitance Bridge"=w488:refnum<class "Instrument.CBridge.lvclass">)
        n183 = call-dynamic "Get Capacitance.vi"("error in (no error)"=w482, "Instrument.CBridge in"=w488) -> ("error out"=w487:errorcluster, "Capacitance (pF)"=w478:dbl, "Instrument.CBridge out"=w479:refnum<class "Instrument.CBridge.lvclass">)  [unwired: 7 in]
        n184 = call <userlib>:"Write Dictionary Element.vi"("error in (no error)"=w487, "value"=w478, "key"="Capacitance", "Control Experiment in"=w486) -> ("error out"=w481:errorcluster, "Control Experiment out"=w483:refnum<class "Control Experiment.lvclass">)  [unwired: 6 in]
        n185 = Bundle By Name(cluster=w485, "Instruments.Capacitance Bridge"=w479, "C.E."=w483) -> (w484:T6)
        n186 = call <vilib>:"Add State(s) to Queue__jki_lib_state_machine.vi"("State(s) in (\"\")"=w490) -> ("States Out"=w489:string)  [unwired: 14 in]
      }
      frame "Measure: Lockin" {
        # "Template Separator\n(You can make a copy of, or modify, this frame)"
        n187 = Unbundle By Name(w503) -> ("C.E."=w502:refnum<class "Control Experiment.lvclass">, "Instruments.Lockin"=w505:refnum<class "Instrument.Lockin.lvclass">)
        n188 = call <userlib>:"waitForNewResults.vi"("error in (no error)"=w506, "Instrument.Lockin in"=w505) -> ("error out"=w500:errorcluster, "Results (Dictionary)"=w494:cluster{"key":string, "value":dbl}[], "Instrument.Lockin out"=w498:refnum<class "Instrument.Lockin.lvclass">)  [unwired: 7 in]
        n189 = call <userlib>:"Parse Results (all).vi"("Type"=Results_Type--Enum."Y", "Results (Dictionary)"=w494) -> ("Data"=w492:dbl[])  [unwired: 6 in, 3 out]
        n190 = call <userlib>:"Parse Results (all).vi"("Type"=Results_Type--Enum."Mean", "Results (Dictionary)"=w494) -> ("Data"=w491:dbl[])  [unwired: 6 in, 3 out]
        n191 = call <userlib>:"Parse Results (all).vi"("Type"=Results_Type--Enum."X", "Results (Dictionary)"=w494) -> ("Data"=w496:dbl[])  [unwired: 6 in, 3 out]
        n192 = for {
          tunnel: w496 -> [w524] mode=indexing
          tunnel: w492 -> [w519] mode=indexing
          tunnel: w500 -> [w518]
          tunnel: [w515] -> w499
          shift-right: [w516] -> w501
          shift-left: w502 -> [w527]
          tunnel: w491 -> [w511] mode=indexing
          i -> [w530]
          n193 = Increment(x=w530) -> (x+1=w514:i32)
          n194 = Format Into String(format string="X%d" ("wavenames"), error in=w518, w514) -> (resulting string=w526:string, error out=w522:errorcluster)  [unwired: 1 in]
          n195 = call <userlib>:"Append Dictionary Element.vi"("error in (no error)"=w522, "value"=w524, "key"=w526, "Control Experiment in"=w527) -> ("error out"=w521:errorcluster, "Control Experiment out"=w523:refnum<class "Control Experiment.lvclass">)  [unwired: 6 in]
          n196 = Format Into String(format string="Y%d" ("wavenames"), error in=w521, w514) -> (resulting string=w525:string, error out=w520:errorcluster)  [unwired: 1 in]
          n197 = call <userlib>:"Append Dictionary Element.vi"("error in (no error)"=w520, "value"=w519, "key"=w525, "Control Experiment in"=w523) -> ("error out"=w510:errorcluster, "Control Experiment out"=w517:refnum<class "Control Experiment.lvclass">)  [unwired: 6 in]
          n198 = Format Into String(format string="Mean%d" ("wavenames"), error in=w510, w514) -> (resulting string=w512:string, error out=w509:errorcluster)  [unwired: 1 in]
          n199 = call <userlib>:"Append Dictionary Element.vi"("error in (no error)"=w509, "value"=w511, "key"=w512, "Control Experiment in"=w517) -> ("error out"=w515:errorcluster, "Control Experiment out"=w516:refnum<class "Control Experiment.lvclass">)  [unwired: 6 in]
        }
        n200 = Bundle By Name(cluster=w503, "Instruments.Lockin"=w498, "Results (Dictionary)"=w494, "C.E."=w501) -> (w504:T6)
        n201 = call <vilib>:"Add State(s) to Queue__jki_lib_state_machine.vi"("State(s) in (\"\")"=w508) -> ("States Out"=w507:string)  [unwired: 14 in]
      }
      frame "Measure: Time" {
        # "Your code here.\n(You can make a copy of, or modify, this frame)"
        n202 = Unbundle By Name(w537) -> ("C.E."=w536:refnum<class "Control Experiment.lvclass">)
        n203 = Get Date/Time In Seconds() -> (seconds since 1Jan1904=w539:timestamp)
        n204 = To Double Precision Float(number=w539) -> (double precision float=w534:dbl)
        n205 = call <userlib>:"Write Dictionary Element.vi"("error in (no error)"=w533, "value"=w534, "key"="Time", "Control Experiment in"=w536) -> ("error out"=w532:errorcluster, "Control Experiment out"=w535:refnum<class "Control Experiment.lvclass">)  [unwired: 6 in]
        n206 = Bundle By Name(cluster=w537, "C.E."=w535) -> (w538:T6)
        n207 = call <vilib>:"Add State(s) to Queue__jki_lib_state_machine.vi"("State(s) in (\"\")"=w541) -> ("States Out"=w540:string)  [unwired: 14 in]
      }
      frame "---------- File ----------" {
        # "Template Separator\n(You can make a copy of, or modify, this frame)"
        n208 = call <vilib>:"Add State(s) to Queue__jki_lib_state_machine.vi"("State(s) in (\"\")"=w545) -> ("States Out"=w544:string)  [unwired: 14 in]
      }
      frame "File: Configure" {
        # "Template Separator\n(You can make a copy of, or modify, this frame)"
        n209 = call <vilib>:"Add State(s) to Queue__jki_lib_state_machine.vi"("State(s) in (\"\")"=w549) -> ("States Out"=w548:string)  [unwired: 14 in]
      }
      frame "File: Save" {
        # "Template Separator\n(You can make a copy of, or modify, this frame)"
        n210 = Unbundle By Name(w552) -> ("C.E."=w557:refnum<class "Control Experiment.lvclass">, "Execution:State"=w554:T7)
        n211 = call <userlib>:"Exec State to Append.vi"("Execution:State"=w554) -> ("append?"=w553:bool)  [unwired: 2 in]
        n212 = call <userlib>:"Save Transport TDMS File.vi"("error in (no error)"=w555, "append?"=w553, "Control Experiment in"=w557) -> ("error out"=w556:errorcluster, "Control Experiment out"=w550:refnum<class "Control Experiment.lvclass">)  [unwired: 7 in]
        n213 = Bundle By Name(cluster=w552, "C.E."=w550) -> (w551:T6)
        n214 = call <vilib>:"Add State(s) to Queue__jki_lib_state_machine.vi"("State(s) in (\"\")"=w559) -> ("States Out"=w558:string)  [unwired: 14 in]
      }
    }
  }
  "error out" <- w2
  n215 = Unbundle By Name(w4) -> ("Transport"=→"Transport.lvclass":refnum<class "Transport.lvclass">)
